vi "M9300A_setall.vi"(7 "resource string":string="PXI0::8-0.0::INSTR", 8 "error in (no error)":errorcluster {"code" format="%.0x"}, 11 "Port setting":T1={"Ch1"=TRUE, "Ch2"=FALSE, "Ch3"=FALSE, "Ch4"=FALSE, "Ch5"=FALSE, "backplane out"=TRUE, "10MHz out"=FALSE, "OCXO out"=FALSE, "bp Ref"=TRUE, "External Ref"=FALSE}) -> (0 "error out":errorcluster {"code" format="%.0x"})   [LabVIEW 2023]
uses:
  Program Files (x86)/Agilent/M938x/LabVIEW Driver/20xx/Agilent M9300/Agilent M9300.lvlib
panel:
  out "bp ref":bool=TRUE
  out "OCXO":bool
  out "Ext Ref":bool
  out "10MHz":bool
  out "back out":bool=TRUE
  out "ch4":bool
  out "ch5":bool
  out "ch3":bool
  out "ch2":bool
  out "ch1":bool=TRUE
  # "Check to make sure the chassis clocked is set to the M9300A, the M9300A is turned on"
  # "Status"
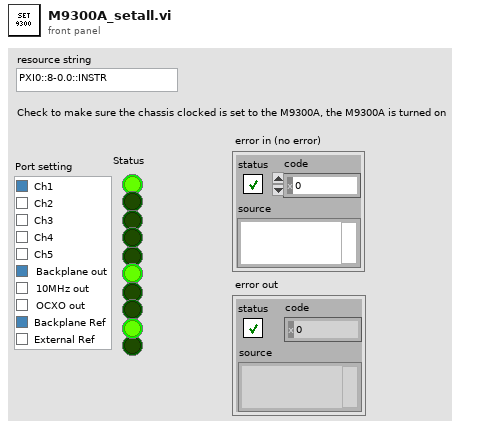
[diagram p1: front panel]
types:
  T1 = cluster{"Ch1":bool, "Ch2":bool, "Ch3":bool, "Ch4":bool, "Ch5":bool, "backplane out":bool, "10MHz out":bool, "OCXO out":bool, "bp Ref":bool, "External Ref":bool}
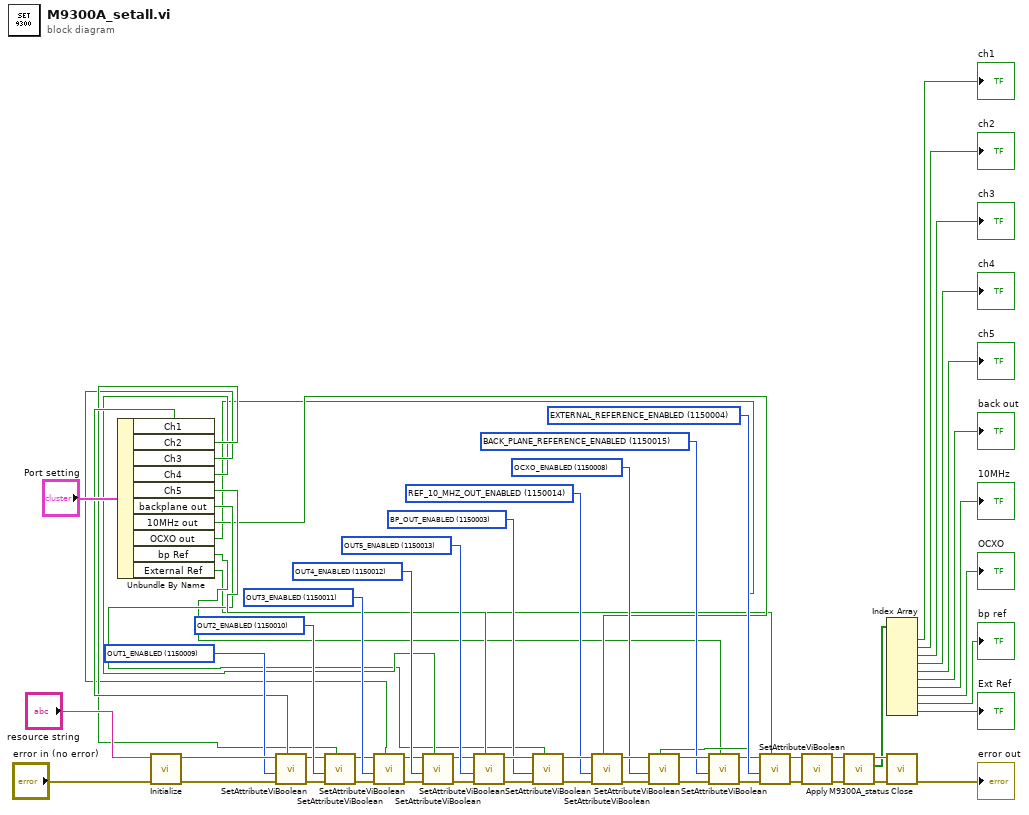
[diagram p0: block diagram]
diagram:
  w27 = u32 1150015 items=["BACK_PLANE_REFERENCE_ENABLED"=1150015, "BP_OUT_ENABLED"=1150003, "EXTERNAL_REFERENCE_ENABLED"=1150004, "NONVOLATILE_ENABLE_INSTRUMENT_CAL_WARNINGS"=1150029, "NONVOLATILE_ENABLE_MODULE_CAL_WARNINGS"=1150028, "NONVOLATILE_ENABLE_PERIODIC_CAL"=1150027, "OCXO_ENABLED"=1150008, "OUT1_ENABLED"=1150009, "OUT2_ENABLED"=1150010, "OUT3_ENABLED"=1150011, "OUT4_ENABLED"=1150012, "OUT5_ENABLED"=1150013, "PROGRAMMABLE_TRIGGER_ENABLED"=1150033, "REF_10_MHZ_OUT_ENABLED"=1150014, "SIMULATE"=1050005, "TRACE_ENABLED"=1150002] ("AttributeID")
  w32 = u32 1150004 items=["BACK_PLANE_REFERENCE_ENABLED"=1150015, "BP_OUT_ENABLED"=1150003, "EXTERNAL_REFERENCE_ENABLED"=1150004, "NONVOLATILE_ENABLE_INSTRUMENT_CAL_WARNINGS"=1150029, "NONVOLATILE_ENABLE_MODULE_CAL_WARNINGS"=1150028, "NONVOLATILE_ENABLE_PERIODIC_CAL"=1150027, "OCXO_ENABLED"=1150008, "OUT1_ENABLED"=1150009, "OUT2_ENABLED"=1150010, "OUT3_ENABLED"=1150011, "OUT4_ENABLED"=1150012, "OUT5_ENABLED"=1150013, "PROGRAMMABLE_TRIGGER_ENABLED"=1150033, "REF_10_MHZ_OUT_ENABLED"=1150014, "SIMULATE"=1050005, "TRACE_ENABLED"=1150002] ("AttributeID")
  w33 = u32 1150008 items=["BACK_PLANE_REFERENCE_ENABLED"=1150015, "BP_OUT_ENABLED"=1150003, "EXTERNAL_REFERENCE_ENABLED"=1150004, "NONVOLATILE_ENABLE_INSTRUMENT_CAL_WARNINGS"=1150029, "NONVOLATILE_ENABLE_MODULE_CAL_WARNINGS"=1150028, "NONVOLATILE_ENABLE_PERIODIC_CAL"=1150027, "OCXO_ENABLED"=1150008, "OUT1_ENABLED"=1150009, "OUT2_ENABLED"=1150010, "OUT3_ENABLED"=1150011, "OUT4_ENABLED"=1150012, "OUT5_ENABLED"=1150013, "PROGRAMMABLE_TRIGGER_ENABLED"=1150033, "REF_10_MHZ_OUT_ENABLED"=1150014, "SIMULATE"=1050005, "TRACE_ENABLED"=1150002] ("AttributeID")
  w34 = u32 1150014 items=["BACK_PLANE_REFERENCE_ENABLED"=1150015, "BP_OUT_ENABLED"=1150003, "EXTERNAL_REFERENCE_ENABLED"=1150004, "NONVOLATILE_ENABLE_INSTRUMENT_CAL_WARNINGS"=1150029, "NONVOLATILE_ENABLE_MODULE_CAL_WARNINGS"=1150028, "NONVOLATILE_ENABLE_PERIODIC_CAL"=1150027, "OCXO_ENABLED"=1150008, "OUT1_ENABLED"=1150009, "OUT2_ENABLED"=1150010, "OUT3_ENABLED"=1150011, "OUT4_ENABLED"=1150012, "OUT5_ENABLED"=1150013, "PROGRAMMABLE_TRIGGER_ENABLED"=1150033, "REF_10_MHZ_OUT_ENABLED"=1150014, "SIMULATE"=1050005, "TRACE_ENABLED"=1150002] ("AttributeID")
  w35 = u32 1150003 items=["BACK_PLANE_REFERENCE_ENABLED"=1150015, "BP_OUT_ENABLED"=1150003, "EXTERNAL_REFERENCE_ENABLED"=1150004, "NONVOLATILE_ENABLE_INSTRUMENT_CAL_WARNINGS"=1150029, "NONVOLATILE_ENABLE_MODULE_CAL_WARNINGS"=1150028, "NONVOLATILE_ENABLE_PERIODIC_CAL"=1150027, "OCXO_ENABLED"=1150008, "OUT1_ENABLED"=1150009, "OUT2_ENABLED"=1150010, "OUT3_ENABLED"=1150011, "OUT4_ENABLED"=1150012, "OUT5_ENABLED"=1150013, "PROGRAMMABLE_TRIGGER_ENABLED"=1150033, "REF_10_MHZ_OUT_ENABLED"=1150014, "SIMULATE"=1050005, "TRACE_ENABLED"=1150002] ("AttributeID")
  w53 = u32 1150013 items=["BACK_PLANE_REFERENCE_ENABLED"=1150015, "BP_OUT_ENABLED"=1150003, "EXTERNAL_REFERENCE_ENABLED"=1150004, "NONVOLATILE_ENABLE_INSTRUMENT_CAL_WARNINGS"=1150029, "NONVOLATILE_ENABLE_MODULE_CAL_WARNINGS"=1150028, "NONVOLATILE_ENABLE_PERIODIC_CAL"=1150027, "OCXO_ENABLED"=1150008, "OUT1_ENABLED"=1150009, "OUT2_ENABLED"=1150010, "OUT3_ENABLED"=1150011, "OUT4_ENABLED"=1150012, "OUT5_ENABLED"=1150013, "PROGRAMMABLE_TRIGGER_ENABLED"=1150033, "REF_10_MHZ_OUT_ENABLED"=1150014, "SIMULATE"=1050005, "TRACE_ENABLED"=1150002] ("AttributeID")
  w54 = u32 1150012 items=["BACK_PLANE_REFERENCE_ENABLED"=1150015, "BP_OUT_ENABLED"=1150003, "EXTERNAL_REFERENCE_ENABLED"=1150004, "NONVOLATILE_ENABLE_INSTRUMENT_CAL_WARNINGS"=1150029, "NONVOLATILE_ENABLE_MODULE_CAL_WARNINGS"=1150028, "NONVOLATILE_ENABLE_PERIODIC_CAL"=1150027, "OCXO_ENABLED"=1150008, "OUT1_ENABLED"=1150009, "OUT2_ENABLED"=1150010, "OUT3_ENABLED"=1150011, "OUT4_ENABLED"=1150012, "OUT5_ENABLED"=1150013, "PROGRAMMABLE_TRIGGER_ENABLED"=1150033, "REF_10_MHZ_OUT_ENABLED"=1150014, "SIMULATE"=1050005, "TRACE_ENABLED"=1150002] ("AttributeID")
  w55 = u32 1150011 items=["BACK_PLANE_REFERENCE_ENABLED"=1150015, "BP_OUT_ENABLED"=1150003, "EXTERNAL_REFERENCE_ENABLED"=1150004, "NONVOLATILE_ENABLE_INSTRUMENT_CAL_WARNINGS"=1150029, "NONVOLATILE_ENABLE_MODULE_CAL_WARNINGS"=1150028, "NONVOLATILE_ENABLE_PERIODIC_CAL"=1150027, "OCXO_ENABLED"=1150008, "OUT1_ENABLED"=1150009, "OUT2_ENABLED"=1150010, "OUT3_ENABLED"=1150011, "OUT4_ENABLED"=1150012, "OUT5_ENABLED"=1150013, "PROGRAMMABLE_TRIGGER_ENABLED"=1150033, "REF_10_MHZ_OUT_ENABLED"=1150014, "SIMULATE"=1050005, "TRACE_ENABLED"=1150002] ("AttributeID")
  w56 = u32 1150010 items=["BACK_PLANE_REFERENCE_ENABLED"=1150015, "BP_OUT_ENABLED"=1150003, "EXTERNAL_REFERENCE_ENABLED"=1150004, "NONVOLATILE_ENABLE_INSTRUMENT_CAL_WARNINGS"=1150029, "NONVOLATILE_ENABLE_MODULE_CAL_WARNINGS"=1150028, "NONVOLATILE_ENABLE_PERIODIC_CAL"=1150027, "OCXO_ENABLED"=1150008, "OUT1_ENABLED"=1150009, "OUT2_ENABLED"=1150010, "OUT3_ENABLED"=1150011, "OUT4_ENABLED"=1150012, "OUT5_ENABLED"=1150013, "PROGRAMMABLE_TRIGGER_ENABLED"=1150033, "REF_10_MHZ_OUT_ENABLED"=1150014, "SIMULATE"=1050005, "TRACE_ENABLED"=1150002] ("AttributeID")
  w57 = u32 1150009 items=["BACK_PLANE_REFERENCE_ENABLED"=1150015, "BP_OUT_ENABLED"=1150003, "EXTERNAL_REFERENCE_ENABLED"=1150004, "NONVOLATILE_ENABLE_INSTRUMENT_CAL_WARNINGS"=1150029, "NONVOLATILE_ENABLE_MODULE_CAL_WARNINGS"=1150028, "NONVOLATILE_ENABLE_PERIODIC_CAL"=1150027, "OCXO_ENABLED"=1150008, "OUT1_ENABLED"=1150009, "OUT2_ENABLED"=1150010, "OUT3_ENABLED"=1150011, "OUT4_ENABLED"=1150012, "OUT5_ENABLED"=1150013, "PROGRAMMABLE_TRIGGER_ENABLED"=1150033, "REF_10_MHZ_OUT_ENABLED"=1150014, "SIMULATE"=1050005, "TRACE_ENABLED"=1150002] ("AttributeID")
  n1 = Unbundle By Name("Port setting") -> ("Ch1"=w10:bool, "Ch2"=w9:bool, "Ch3"=w8:bool, "Ch4"=w7:bool, "Ch5"=w6:bool, "backplane out"=w5:bool, "10MHz out"=w4:bool, "OCXO out"=w3:bool, "bp Ref"=w2:bool, "External Ref"=w1:bool)
  n2 = call "Initialize.vi"("error in (no error)"="error in (no error)", "resource string"="resource string") -> ("error out"=w59:errorcluster, "instrument handle out"=w58:refnum<k15>)  [unwired: 8 in]
  n3 = call "SetAttributeViBoolean.vi"("AttributeValue (Off)"=w10, "error in (no error)"=w59, "AttributeID"=w57, "instrument handle"=w58) -> ("error out"=w51:errorcluster, "instrument handle out"=w52:refnum<k15>)  [unwired: 6 in]
  n4 = call "SetAttributeViBoolean.vi"("AttributeValue (Off)"=w9, "error in (no error)"=w51, "AttributeID"=w56, "instrument handle"=w52) -> ("error out"=w49:errorcluster, "instrument handle out"=w50:refnum<k15>)  [unwired: 6 in]
  n5 = call "SetAttributeViBoolean.vi"("AttributeValue (Off)"=w8, "error in (no error)"=w49, "AttributeID"=w55, "instrument handle"=w50) -> ("error out"=w48:errorcluster, "instrument handle out"=w47:refnum<k15>)  [unwired: 6 in]
  n6 = call "SetAttributeViBoolean.vi"("AttributeValue (Off)"=w7, "error in (no error)"=w48, "AttributeID"=w54, "instrument handle"=w47) -> ("error out"=w45:errorcluster, "instrument handle out"=w46:refnum<k15>)  [unwired: 6 in]
  n7 = call "SetAttributeViBoolean.vi"("AttributeValue (Off)"=w6, "error in (no error)"=w45, "AttributeID"=w53, "instrument handle"=w46) -> ("error out"=w43:errorcluster, "instrument handle out"=w39:refnum<k15>)  [unwired: 6 in]
  n8 = call "SetAttributeViBoolean.vi"("AttributeValue (Off)"=w5, "error in (no error)"=w43, "AttributeID"=w35, "instrument handle"=w39) -> ("error out"=w42:errorcluster, "instrument handle out"=w38:refnum<k15>)  [unwired: 6 in]
  n9 = call "SetAttributeViBoolean.vi"("AttributeValue (Off)"=w4, "error in (no error)"=w42, "AttributeID"=w34, "instrument handle"=w38) -> ("error out"=w41:errorcluster, "instrument handle out"=w37:refnum<k15>)  [unwired: 6 in]
  n10 = call "SetAttributeViBoolean.vi"("AttributeValue (Off)"=w3, "error in (no error)"=w41, "AttributeID"=w33, "instrument handle"=w37) -> ("error out"=w30:errorcluster, "instrument handle out"=w31:refnum<k15>)  [unwired: 6 in]
  n11 = call "SetAttributeViBoolean.vi"("AttributeValue (Off)"=w2, "error in (no error)"=w30, "AttributeID"=w27, "instrument handle"=w31) -> ("error out"=w28:errorcluster, "instrument handle out"=w29:refnum<k15>)  [unwired: 6 in]
  n12 = call "SetAttributeViBoolean.vi"("AttributeValue (Off)"=w1, "error in (no error)"=w28, "AttributeID"=w32, "instrument handle"=w29) -> ("error out"=w40:errorcluster, "instrument handle out"=w36:refnum<k15>)  [unwired: 6 in]
  n13 = call "Apply.vi"("error in (no error)"=w40, "instrument handle"=w36) -> ("error out"=w25:errorcluster, "instrument handle out"=w26:refnum<k15>)  [unwired: 8 in]
  n14 = call "M9300A_status.vi"("error in (no error)"=w25, "instrument handle in"=w26) -> ("error out"=w24:errorcluster, "Status"=w22:bool[], "instrument handle out"=w23:refnum<k15>)  [unwired: 7 in]
  n15 = Index Array(array=w22) -> (element #1=→"ch1":bool, element #2=→"ch2":bool, element #3=→"ch3":bool, element #4=→"ch4":bool, element #5=→"ch5":bool, element #6=→"back out":bool, element #7=→"10MHz":bool, element #8=→"OCXO":bool, element #9=→"bp ref":bool, element #10=→"Ext Ref":bool)  [unwired: 10 in]
  n16 = call "Close.vi"("error in (no error)"=w24, "instrument handle"=w23) -> ("error out"=→"error out":errorcluster)  [unwired: 9 in]
